vi "Validate.vi"(8 "error in (no error)":errorcluster, 11 "AB_UI_Fmwrk_Build in":refnum<class "AB_UI_Frmwk_Build.lvclass">) -> (0 "error out":errorcluster, 3 "AB_UI_Fmwrk_Build out":refnum<class "AB_UI_Frmwk_Build.lvclass">)   [LabVIEW 2020, in "AB_UI_Frmwk_Build.lvclass"]
uses:
  <vilib>/AppBuilder/AB_Classes/Build/UI/AB_UI_Frmwk_Build.lvclass
  <vilib>/AppBuilder/AB_Classes/Build/AB_Build.lvclass
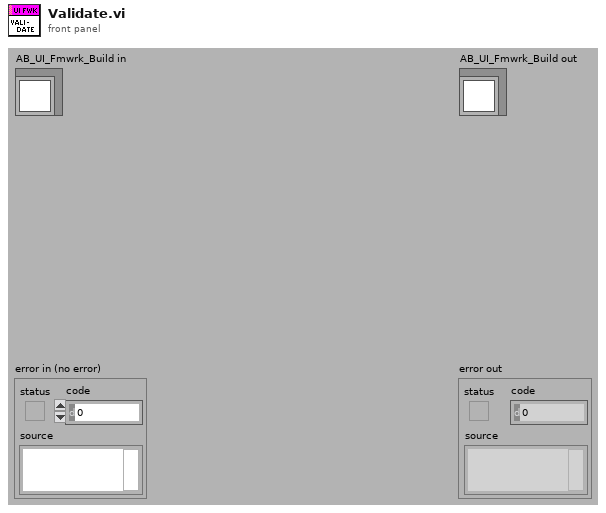
[diagram p1: front panel]
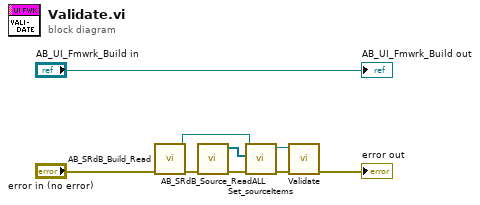
[diagram p0: block diagram]
diagram:
  n1 = call <resource>:"AB_SRdB_Build_Read.vi"("error in (no error)"="error in (no error)") -> ("error out"=w6:errorcluster, "build out"=w8:refnum<class "AB_Build.lvclass">)  [unwired: 9 out]
  n2 = call <resource>:"AB_SRdB_Source_ReadALL.vi"("error in (no error)"=w6) -> ("error out"=w5:errorcluster, "ALL data"=w7:refnum<class "AB_Source.lvclass">[])  [unwired: 9 out]
  n3 = call <vilib>:"Set_sourceItems.vi"("error in (no error)"=w5, "sourceItems"=w7, "Class in"=w8) -> ("error out"=w4:errorcluster, "Class out"=w9:refnum<class "AB_Build.lvclass">)  [unwired: 7 out]
  n4 = call-dynamic "Validate.vi"("error in (no error)"=w4, "Build in"=w9) -> ("error out"=→"error out":errorcluster)  [unwired: 9 out]
  "AB_UI_Fmwrk_Build out" <- "AB_UI_Fmwrk_Build in"
